vi "Configure Power Measurement Statistics.vi"(7 "Statistic Count (10)":i32=10 format="%.0g", 8 "error in (no error)":errorcluster, 9 "Repetition (Single)":i32(ring) items=["Single", "Continuous"], 10 "Instance (1)":i32=1 format="%.0g", 11 "VISA resource name":refnum<visa-resource-name>) -> (0 "error out":errorcluster, 3 "VISA resource name out":refnum<visa-resource-name>)   [LabVIEW 2020, in "Rohde&Schwarz CMXP GPRF.lvlib"]
doc: "Specifies the scope of the measurement.\n\nAttributes:\nRSCMXPGPRF_ATTR_POWER_MEASUREMENT_REPETITION_MODE\nRSCMXPGPRF_ATTR_POWER_MEASUREMENT_COUNT\n\nRemote-control commands:\nCONFigure:GPRF:MEAS<i>:POWer:REPetition\nCONFigure:GPRF:MEAS<i>:POWer:SCOunt"
uses:
  <instrlib>/Rohde&Schwarz CMXP GPRF/Rohde&Schwarz CMXP GPRF.lvlib
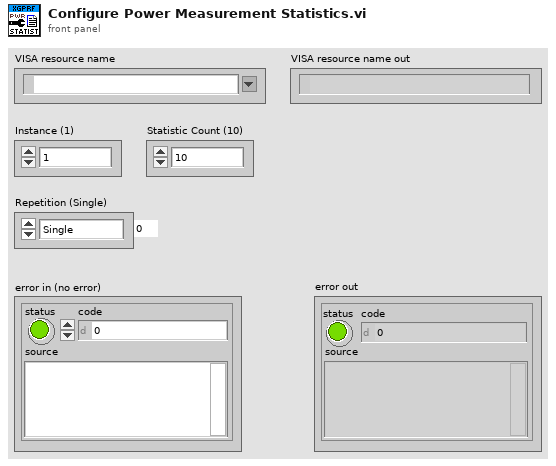
[diagram p1: front panel]
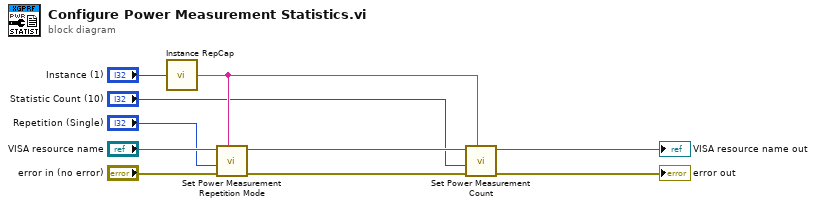
[diagram p0: block diagram]
diagram:
  n1 = call <instrlib>:"Instance RepCap.vi"("Instance in"="Instance (1)") -> ("Instance out"=w10:string)
  n2 = call "Set Power Measurement Repetition Mode"("Repeated Capabilities"=w10, "error in (no error)"="error in (no error)", "Power Measurement Repetition Mode (0 - Single)"="Repetition (Single)", "instrument handle"="VISA resource name") -> ("error out"=w7:errorcluster, "instrument handle out"=w4:refnum<visa-resource-name>)  [unwired: 6 in]
  n3 = call "Set Power Measurement Count"("Repeated Capabilities"=w10, "error in (no error)"=w7, "Power Measurement Count (0)"="Statistic Count (10)", "instrument handle"=w4) -> ("error out"=→"error out":errorcluster, "instrument handle out"=→"VISA resource name out":refnum<visa-resource-name>)  [unwired: 6 in]
